vi "图像测试.vi"(8 "error in":errorcluster, 10 "保留图像？":bool, 11 "Session In":T1="cam0") -> (0 "error out":errorcluster, 1 "数量":i32[](array[numeric]), 2 "大小":dbl[](array[numeric]), 3 "Image Out":T2(plugin-control))   [LabVIEW 2017]
uses:
  <vilib>/userdefined/High Color/IMAQdx.ctl
  <vilib>/vision/NI_Vision_Development_Module.lvlib
  <vilib>/vision/driver/NI_Vision_Acquisition_Software.lvlib
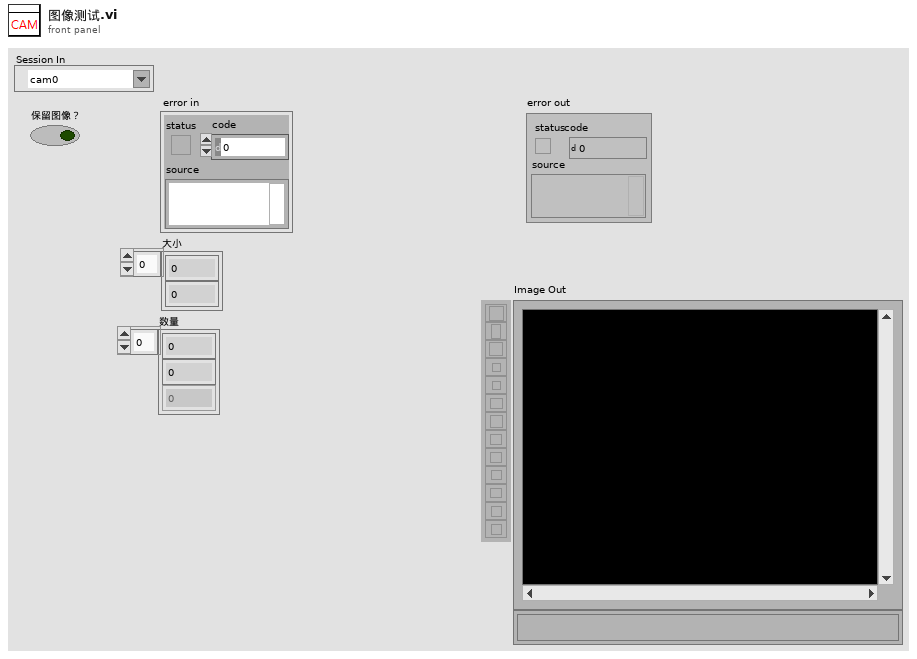
[diagram p1: front panel]
types:
  T1 = typedef "IMAQdx.ctl" = refnum<k21>
  T2 = typedef "IMAQ Image.ctl" = refnum<image>
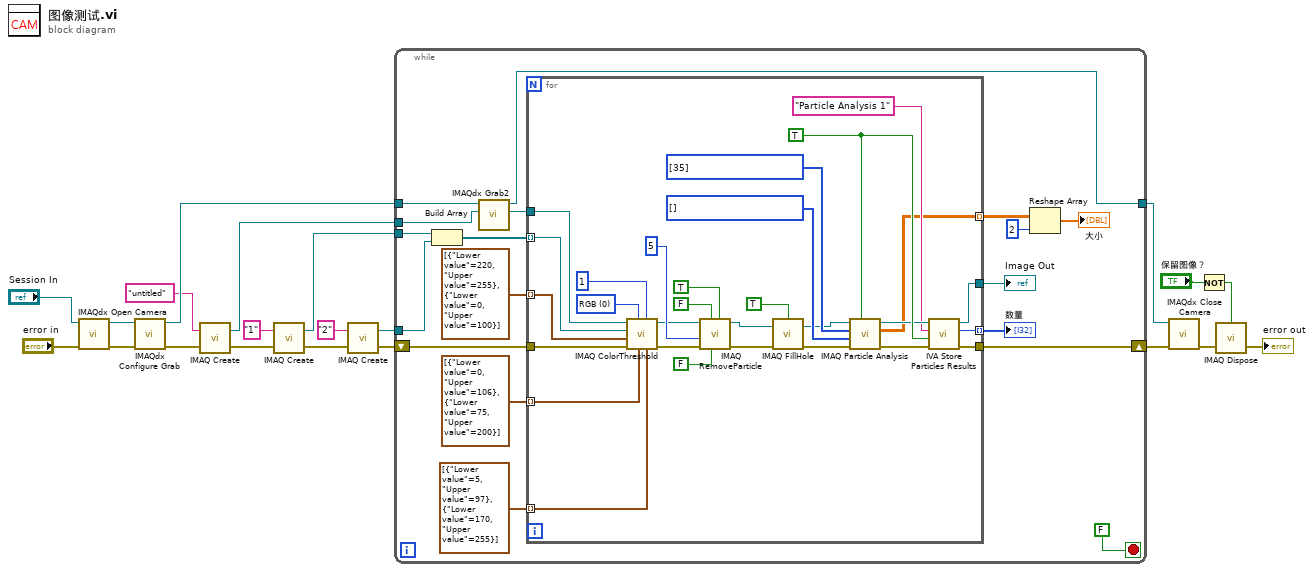
[diagram p0: block diagram]
diagram:
  n1 = call <vilib>:"IMAQdx Open Camera.vi"("error in"="error in", "Session In"="Session In") -> ("error out"=w17:errorcluster, "Session Out"=w16:T1)  [unwired: 8 in]
  n2 = call <vilib>:"IMAQdx Configure Grab.vi"("error in"=w17, "Session In"=w16) -> ("error out"=w14:errorcluster, "Session Out"=w21:T1)  [unwired: 8 in]
  n3 = call "IMAQ Create"("Image Name"="untitled", "error in (no error)"=w14) -> ("New Image"=w19:T2, "error out"=w11:errorcluster)  [unwired: 3 in]
  n4 = call "IMAQ Create"("Image Name"="1", "error in (no error)"=w11) -> ("New Image"=w8:T2, "error out"=w9:errorcluster)  [unwired: 3 in]
  n5 = call "IMAQ Create"("Image Name"="2", "error in (no error)"=w9) -> ("New Image"=w7:T2, "error out"=w6:errorcluster)  [unwired: 3 in]
  n6 = while {
    tunnel: w19 -> [w37]
    tunnel: w8 -> [w29]
    tunnel: w7 -> [w28]
    shift-right: [w23] -> w5
    shift-left: w6 -> [w24]
    tunnel: w21 -> [w39]
    tunnel: [w38] -> w20
    stop <- FALSE stop-if-true
    n7 = Build Array(w29, w28) -> (w36:T2[])
    n8 = call <vilib>:"IMAQdx Grab2.vi"("Image In"=w37, "Session In"=w39) -> ("Image Out"=w30:T2, "Session Out"=w38:T1)  [unwired: 6 in, 2 out]
    n9 = for {
      tunnel: cluster{"Lower value":i32, "Upper value":i32}[] [{"Lower value"=220, "Upper value"=255}, {"Lower value"=0, "Upper value"=100}] -> [w66] mode=indexing
      tunnel: cluster{"Lower value":i32, "Upper value":i32}[] [{"Lower value"=0, "Upper value"=106}, {"Lower value"=75, "Upper value"=200}] -> [w65] mode=indexing
      tunnel: cluster{"Lower value":i32, "Upper value":i32}[] [{"Lower value"=5, "Upper value"=97}, {"Lower value"=170, "Upper value"=255}] -> [w64] mode=indexing
      tunnel: [w46] -> w31 mode=indexing
      tunnel: [w44] -> w27 mode=indexing
      tunnel: w30 -> [w43]
      tunnel: [w45] -> w35
      tunnel: w36 -> [w42] mode=indexing
      tunnel: w24 -> [w41]
      tunnel: [w40] -> w23
      w52 = i32[] [] items=["Center of Mass X", "Center of Mass Y", "First Pixel X", "First Pixel Y", "Bounding Rect Left", "Bounding Rect Top", "Bounding Rect Right", "Bounding Rect Bottom", "Max Feret Diameter Start X", "Max Feret Diameter Start Y", "Max Feret Diameter End X", "Max Feret Diameter End Y", "Max Horiz. Segment Length Left", "Max Horiz. Segment Length Right", "Max Horiz. Segment Length Row", "-", "Bounding Rect Width", "Bounding Rect Height", "Bounding Rect Diagonal", "Perimeter", "Convex Hull Perimeter", "Holes' Perimeter", "Max Feret Diameter", "Equivalent Ellipse Major Axis", "Equivalent Ellipse Minor Axis", "Equivalent Ellipse Minor Axis (Feret)", "Equivalent Rect Long Side", "Equivalent Rect Short Side", "Equivalent Rect Diagonal", "Equivalent Rect Short Side (Feret)", "Average Horiz. Segment Length", "Average Vert. Segment Length", "Hydraulic Radius", "Waddel Disk Diameter", "-", "Area", "Holes' Area", "Particle & Holes' Area", "Convex Hull Area", "Image Area", "-", "Number of Holes", "Number of Horiz. Segments", "Number of Vert. Segments", "-", "Orientation", "Max Feret Diameter Orientation", "-", "% Area/Image Area", "% Area/(Particle & Holes' Area)", "Ratio of Equivalent Ellipse Axes", "Ratio of Equivalent Rect Sides", "-", "Elongation Factor", "Compactness Factor", "Heywood Circularity Factor", "Type Factor", "-", "Sum X", "Sum Y", "Sum XX", "Sum XY", "Sum YY", "Sum XXX", "Sum XXY", "Sum XYY", "Sum YYY", "-", "Moment of Inertia XX", "Moment of Inertia XY", "Moment of Inertia YY", "Moment of Inertia XXX", "Moment of Inertia XXY", "Moment of Inertia XYY", "Moment of Inertia YYY", "Norm. Moment of Inertia XX", "Norm. Moment of Inertia XY", "Norm. Moment of Inertia YY", "Norm. Moment of Inertia XXX", "Norm. Moment of Inertia XXY", "Norm. Moment of Inertia XYY", "Norm. Moment of Inertia YYY", "Hu Moment 1", "Hu Moment 2", "Hu Moment 3", "Hu Moment 4", "Hu Moment 5", "Hu Moment 6", "Hu Moment 7"] ("Real-World Measurements")
      w53 = i32[] [35] items=["Center of Mass X", "Center of Mass Y", "First Pixel X", "First Pixel Y", "Bounding Rect Left", "Bounding Rect Top", "Bounding Rect Right", "Bounding Rect Bottom", "Max Feret Diameter Start X", "Max Feret Diameter Start Y", "Max Feret Diameter End X", "Max Feret Diameter End Y", "Max Horiz. Segment Length Left", "Max Horiz. Segment Length Right", "Max Horiz. Segment Length Row", "-", "Bounding Rect Width", "Bounding Rect Height", "Bounding Rect Diagonal", "Perimeter", "Convex Hull Perimeter", "Holes' Perimeter", "Max Feret Diameter", "Equivalent Ellipse Major Axis", "Equivalent Ellipse Minor Axis", "Equivalent Ellipse Minor Axis (Feret)", "Equivalent Rect Long Side", "Equivalent Rect Short Side", "Equivalent Rect Diagonal", "Equivalent Rect Short Side (Feret)", "Average Horiz. Segment Length", "Average Vert. Segment Length", "Hydraulic Radius", "Waddel Disk Diameter", "-", "Area", "Holes' Area", "Particle & Holes' Area", "Convex Hull Area", "Image Area", "-", "Number of Holes", "Number of Horiz. Segments", "Number of Vert. Segments", "-", "Orientation", "Max Feret Diameter Orientation", "-", "% Area/Image Area", "% Area/(Particle & Holes' Area)", "Ratio of Equivalent Ellipse Axes", "Ratio of Equivalent Rect Sides", "-", "Elongation Factor", "Compactness Factor", "Heywood Circularity Factor", "Type Factor", "-", "Sum X", "Sum Y", "Sum XX", "Sum XY", "Sum YY", "Sum XXX", "Sum XXY", "Sum XYY", "Sum YYY", "-", "Moment of Inertia XX", "Moment of Inertia XY", "Moment of Inertia YY", "Moment of Inertia XXX", "Moment of Inertia XXY", "Moment of Inertia XYY", "Moment of Inertia YYY", "Norm. Moment of Inertia XX", "Norm. Moment of Inertia XY", "Norm. Moment of Inertia YY", "Norm. Moment of Inertia XXX", "Norm. Moment of Inertia XXY", "Norm. Moment of Inertia XYY", "Norm. Moment of Inertia YYY", "Hu Moment 1", "Hu Moment 2", "Hu Moment 3", "Hu Moment 4", "Hu Moment 5", "Hu Moment 6", "Hu Moment 7"] ("Pixel Measurements")
      w50 = TRUE ("Connectivity 4/8 (8)")
      w67 = u16 0 items=["RGB", "HSL", "HSV", "HSI"] ("Color Mode")
      n10 = call "IMAQ ColorThreshold"("Blue or Luma or Val or Inten Range"=w64, "Replace Value"=1, "Green or Sat Range"=w65, "Color Mode"=w67, "error in (no error)"=w41, "Red or Hue Range"=w66, "Image Dst"=w42, "Image Src"=w43) -> ("error out"=w63:errorcluster, "Image Dst Out"=w58:T2)  [unwired: 2 out]
      n11 = call "IMAQ RemoveParticle"("Connectivity 4/8 (8)"=TRUE, "Low Pass/High Pass (Low)"=FALSE, "Square/Hexa (Square)"=FALSE, "error in (no error)"=w63, "Number of Erosion"=5, "Image Src"=w58) -> ("error out"=w57:errorcluster, "Image Dst Out"=w55:T2)  [unwired: 1 in, 3 out]
      n12 = call "IMAQ FillHole"("error in (no error)"=w57, "Image Src"=w55, "Connectivity 4/8 (8)"=TRUE) -> ("error out"=w54:errorcluster, "Image Dst Out"=w51:T2)  [unwired: 1 in, 2 out]
      n13 = call "IMAQ Particle Analysis"("Connectivity 4/8 (8)"=w50, "error in (no error)"=w54, "Real-World Measurements"=w52, "Pixel Measurements"=w53, "Image"=w51) -> ("error out"=w47:errorcluster, "Particle Measurements (Pixels)"=w44:dbl[][], "Image Out (duplicate)"=w49:T2)  [unwired: 4 out]
      n14 = call <vilib>:"IVA Store Particles Results.vi"("error in (no error)"=w47, "Connectivity 4/8 (8)"=w50, "Step Name"="Particle Analysis 1", "Image in"=w49) -> ("error out"=w40:errorcluster, "Number of Particles"=w46:i32, "Image dup"=w45:T2)  [unwired: 5 out]
    }
    "Image Out" <- w35
    "数量" <- w31
    n15 = Reshape Array(w27, 2 ("维数大小")) -> (→"大小":dbl[])
  }
  n16 = call <vilib>:"IMAQdx Close Camera.vi"("error in"=w5, "Session In"=w20) -> ("error out"=w18:errorcluster)  [unwired: 9 in]
  n17 = Not(x="保留图像？") -> (.not. x?=w1:bool)
  n18 = call "IMAQ Dispose"("All Images? (No)"=w1, "error in (no error)"=w18) -> ("error out"=→"error out":errorcluster)  [unwired: 4 in]
